vi "Autonomous Independent.vi"() -> ()   [LabVIEW 2016]
doc: "This VI is called when autonomous begins, and will automatically be terminated when autonomous ends. You can carry out timed or sensor driven robot movement independently without needing to return to the caller."
uses:
  <vilib>/Rock Robotics/WPI/Solenoid/WPI_SolenoidValue.ctl
  <vilib>/Rock Robotics/WPI/Utilities/WPI_GetSetVariantRefNum.vi
  <vilib>/Rock Robotics/Network Tables/NT Read String.vi
  <vilib>/Rock Robotics/Network Tables/NT Write Numeric Array.vi
  <vilib>/Rock Robotics/WPI/RobotDrive/WPI_RobotDriveArcadeDrive_Standard(NoSaturation).vi
  <vilib>/Rock Robotics/WPI/Solenoid/WPI_SolenoidSetEnum.vi
panel:
  out "encodervalue":dbl
  in  "Reset":bool
  out "Current Movement, for debugging":T1 {"Y Joystick Value" scale=1.0..-1.0; "X Joystick Value" scale=-1.0..1.0}
  in  "Array of robot movements":T2(array[cluster])=[{"X Joystick Value"=0.39393939393939403, "Y Joystick Value"=0.0, "Delay (sec)"=1.0, "Movement Name"="turn"}, {"X Joystick Value"=-0.3737373737373737, "Y Joystick Value"=0.0, "Delay (sec)"=1.0, "Movement Name"="turn back"}] {"Y Joystick Value" scale=1.0..-1.0; "X Joystick Value" scale=-1.0..1.0}
  # "Be sure to right-click and choose Data Operations>>Make Current Value default if you want to save the array values with the VI"
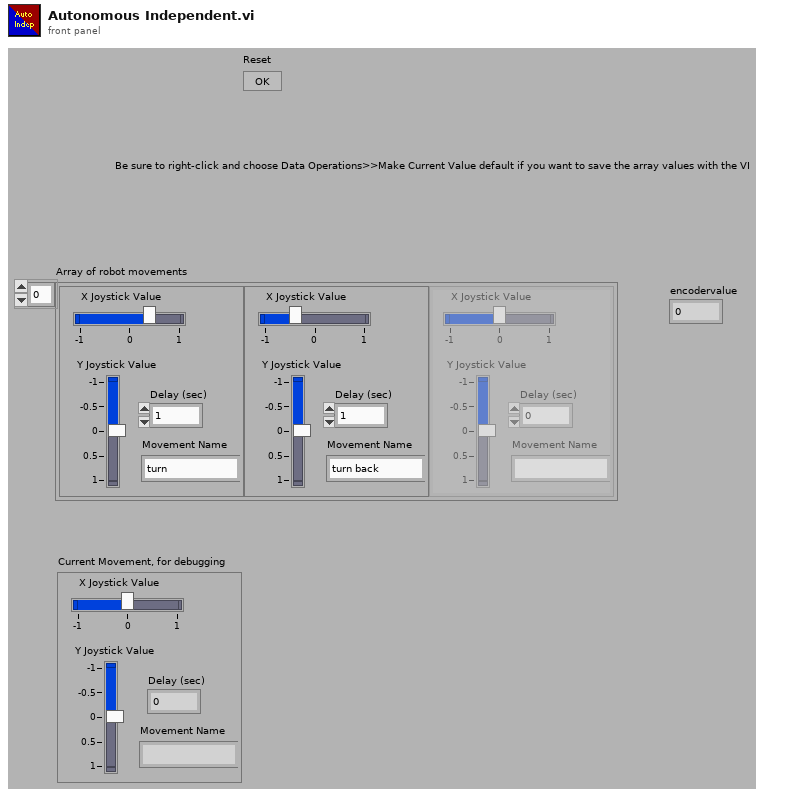
[diagram p1: front panel]
types:
  T1 = cluster{"X Joystick Value":dbl, "Y Joystick Value":dbl, "Delay (sec)":dbl, "Movement Name":string}
  T2 = cluster{"X Joystick Value":dbl, "Y Joystick Value":dbl, "Delay (sec)":dbl, "Movement Name":string}[]
  T3 = typedef "WPI_JoystickDevRef.ctl" = cluster{"Device":T4}
  T4 = typedef "WPI_JoystickDeviceEnum.ctl" = enum16{"USB 0", "USB 1", "USB 2", "USB 3", "USB 4", "USB 5"}
  T5 = typedef "WPI_EncoderDevRef.ctl" = cluster{"DevStatus":errorcluster, "EncoderIndex":T6, "CounterIndex":T7, "DistancePerCount":dbl, "Decoding Type":T8}
  T6 = typedef "FPGA_EncoderIdx.ctl" = enum8{"Enc 0", "Enc 1", "Enc 2", "Enc 3", "Enc 4", "Enc 5", "Enc 6", "Enc 7", "Invalid"}
  T7 = typedef "FPGA_CounterCtrSystemIndex.ctl" = enum8{"Ctr 0", "Ctr 1", "Ctr 2", "Ctr 3", "Ctr 4", "Ctr 5", "Ctr 6", "Ctr 7", "Invalid"}
  T8 = typedef "WPI_EncoderType.ctl" = enum16{"1x", "2x", "4x"}
  T9 = typedef "WPI_GyroDevRef.ctl" = cluster{"DevStatus":errorcluster, "Analog Channel":T10, "Offset":dbl, "Gain (VoltsPerDegree/Second)":dbl, "Gyro Type":enum16{"Analog", "XRS450"}, "Handle":i32, "SPI Bus":T11, "Device Found":bool, "Sample Rate":dbl, "Calibrate On Open":bool}
  T10 = typedef "FPGA_AIChannel.ctl" = enum8{"AI 0", "AI 1", "AI 2", "AI 3", "AI MXP 0", "AI MXP 1", "AI MXP 2", "AI MXP 3", "Invalid"}
  T11 = typedef "spi_bus.ctl" = enum16{"SPI On-Board, CS0", "SPI On-Board, CS1", "SPI On-Board, CS2", "SPI On-Board, CS3", "SPI MXP", "Invalid"}
  T12 = typedef "WPI_RobotDriveDevRef.ctl" = cluster{"DevStatus":errorcluster, "Motors[]":T13[], "Square Inputs":bool, "Max Output":dbl}
  T13 = typedef "WPI_MotorControlDeviceRef.ctl" = cluster{"DeviceStatus":errorcluster, "Type":T14, "PWM":cluster{"PWM Channel":T15, "DeadBand":T16}, "CAN":cluster{"Device Number":u8, "SetOutput VI Ref":variant, "GetOutput VI Ref":variant, "Enable VI Ref":variant, "Disable VI Ref":variant, "Data":variant}, "Invert":bool}
  T14 = typedef "WPI_MotorControlType.ctl" = enum16{"PWM", "CAN"}
  T15 = typedef "FPGA_DIOPWMChannel.ctl" = enum8{"PWM 0", "PWM 1", "PWM 2", "PWM 3", "PWM 4", "PWM 5", "PWM 6", "PWM 7", "PWM 8", "PWM 9", "PWM MXP 0", "PWM MXP 1", "PWM MXP 2", "PWM MXP 3", "PWM MXP 4", "PWM MXP 5", "PWM MXP 6", "PWM MXP 7", "PWM MXP 8", "PWM MXP 9", "Invalid"}
  T16 = typedef "WPI_PWMDeadband.ctl" = cluster{"Name":string, "maxPositivePwm":i32, "minPositivePwm":i32, "centerPwm":i32, "maxNegativePwm":i32, "minNegativePwm":i32, "angularRange":u16}
  T17 = typedef "WPI_SolenoidValue.ctl" = enum16{"Off", "On", "Forward", "Reverse"}
  T18 = typedef "WPI_SolenoidDevRef.ctl" = cluster{"DevStatus":errorcluster, "Pneumatics Control Module":u8, "Forward Solenoid Channel":T19, "Reverse Solenoid Channel":T19}
  T19 = typedef "WPI_SolenoidChannel.ctl" = enum8{"Solenoid 0", "Solenoid 1", "Solenoid 2", "Solenoid 3", "Solenoid 4", "Solenoid 5", "Solenoid 6", "Solenoid 7", "Invalid"}
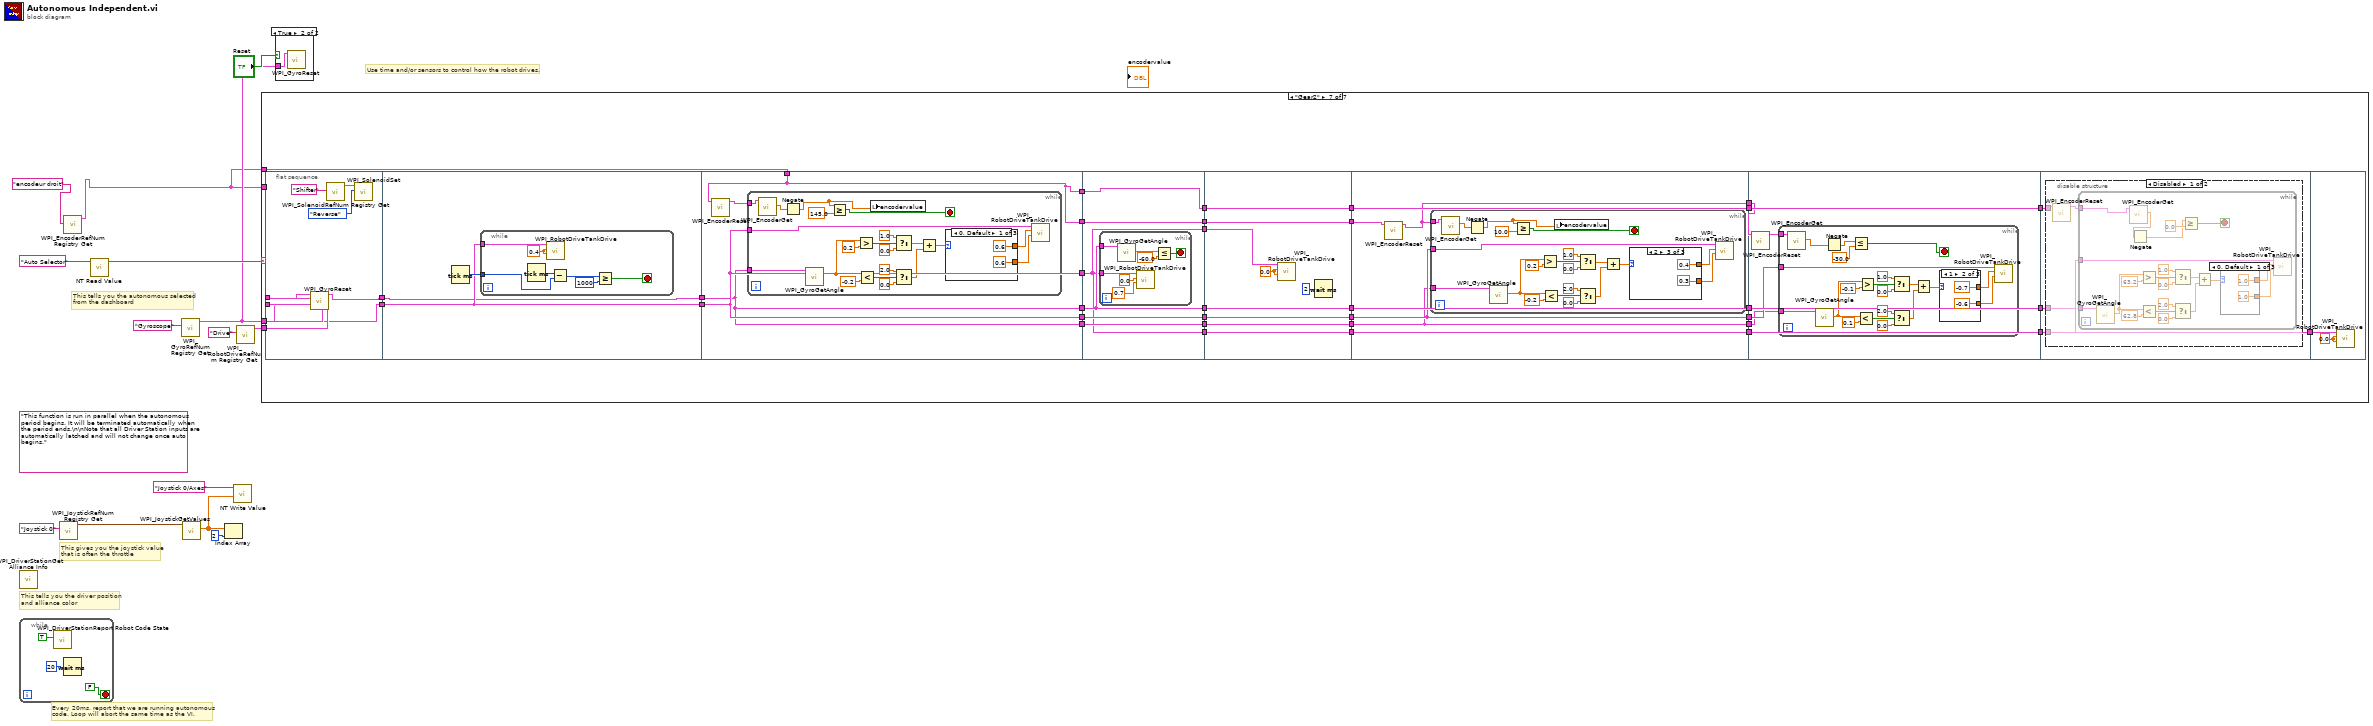
[diagram p0: block diagram]
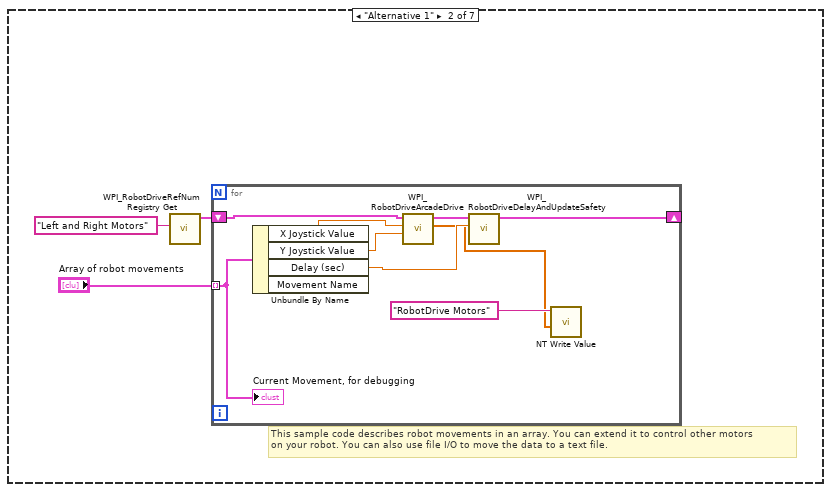
[diagram p4: hidden frame]
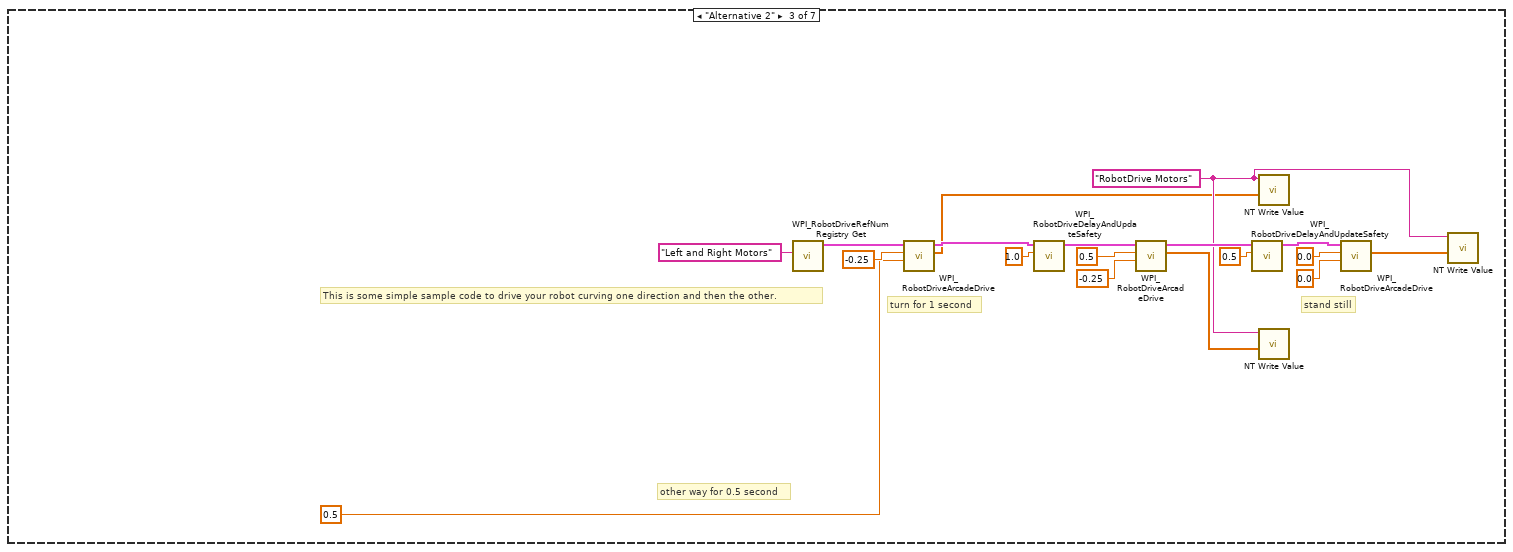
[diagram p5: hidden frame]
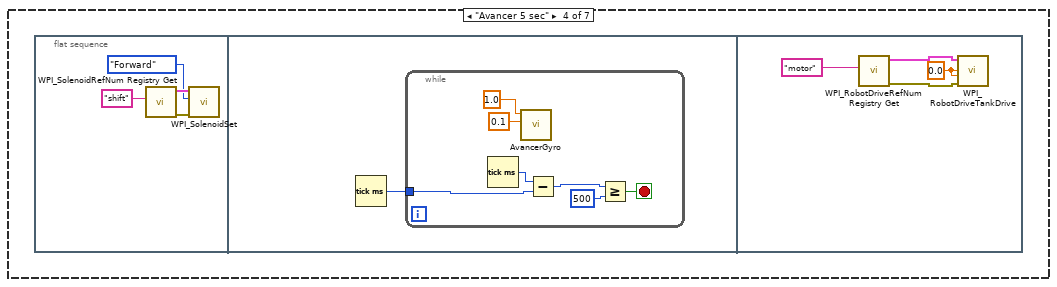
[diagram p6: hidden frame]
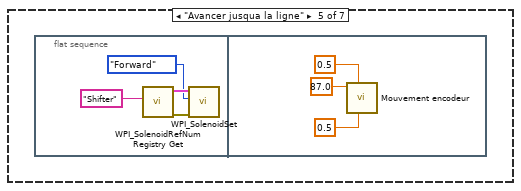
[diagram p7: hidden frame]
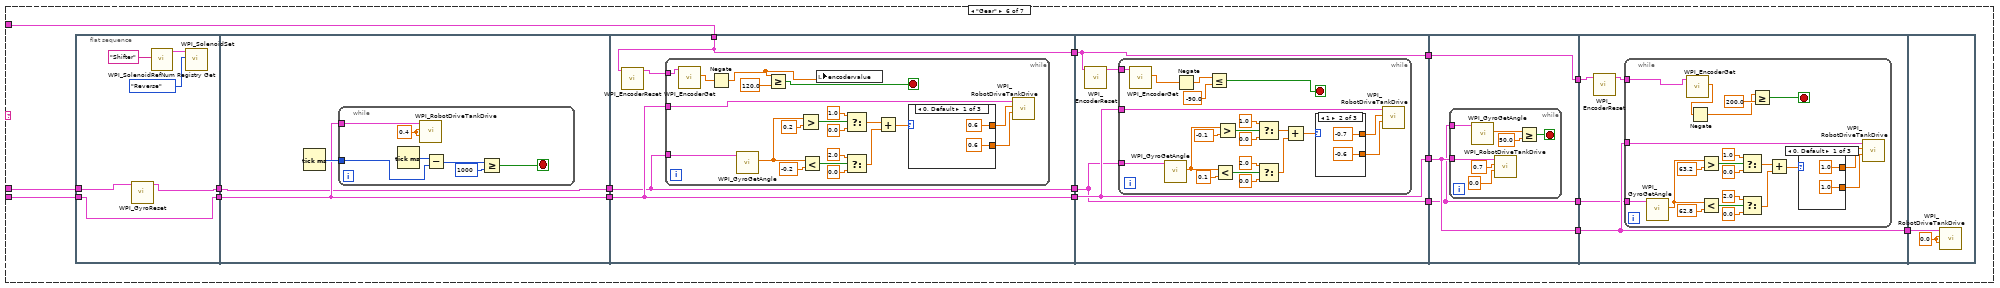
[diagram p8: hidden frame]
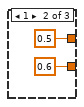
[diagram p9: hidden frame]
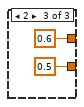
[diagram p10: hidden frame]
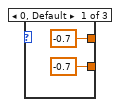
[diagram p11: hidden frame]
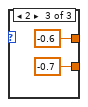
[diagram p12: hidden frame]
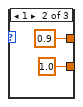
[diagram p13: hidden frame]
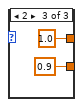
[diagram p14: hidden frame]
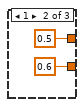
[diagram p15: hidden frame]
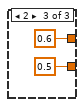
[diagram p16: hidden frame]
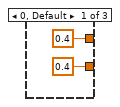
[diagram p17: hidden frame]
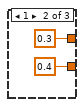
[diagram p18: hidden frame]
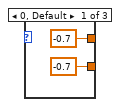
[diagram p19: hidden frame]
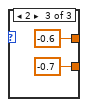
[diagram p20: hidden frame]
diagram:
  (unwired) "This function is run in parallel when the autonomous period begins. It will be terminated automatically when the period ends.\n\nNote that all Driver Station inputs are automatically latched and will not change once auto begins."
  # "This tells you the autonomous selected\nfrom the dashboard"
  # "Every 20ms, report that we are running autonomous\ncode. Loop will abort the same time as the VI."
  # "This gives you the joystick value\nthat is often the throttle"
  # "Use time and/or sensors to control how the robot drives."
  # "This tells you the driver position\nand alliance color"
  n1 = call <vilib>:"WPI_DriverStationGet Alliance Info.vi"() -> ()  [unwired: 12 out]
  n2 = while {
    stop <- FALSE stop-if-true
    n3 = call <vilib>:"WPI_DriverStationReport Robot Code State.vi"("Autonomous"=TRUE) -> ()  [unwired: 10 in, 1 out]
    n4 = Wait (ms)(milliseconds to wait=u32 20) -> ()  [unwired: 1 out]
  }
  n5 = call <vilib>:"WPI_JoystickRefNum Registry Get.vi"("refnum name"="Joystick 0") -> ("JoystickDevRef"=w13:T3)  [unwired: 1 in, 9 out]
  n6 = call <vilib>:"WPI_EncoderRefNum Registry Get.vi"("refnum name"="encodeur droit") -> ("EncoderDevRef"=w1:T5)  [unwired: 9 in, 1 out]
  n7 = call-poly <vilib>:"NT Read Value.vi"("Name"="Auto Selector") -> ("String"=w8:string)  [unwired: 9 in, 1 out]
  n8 = call <vilib>:"WPI_GyroRefNum Registry Get.vi"("refnum name"="Gyroscope") -> ("GyroDevRef"=w3:T9)  [unwired: 9 in, 1 out]
  n9 = call <vilib>:"WPI_JoystickGetValues.vi"("JoystickDevRef"=w13) -> ("Axes"=w10:dbl[])  [unwired: 6 in, 4 out]
  n10 = Index Array(array=w10, index=2) -> ()  [unwired: 1 out]
  n11 = call-poly <vilib>:"NT Write Value.vi"("Numeric Array"=w10, "Name"="Joystick 0/Axes") -> ()  [unwired: 9 in, 1 out]
  n12 = call <vilib>:"WPI_RobotDriveRefNum Registry Get.vi"("refnum name"="Drive") -> ("RobotDriveDevRef"=w6:T12)  [unwired: 9 in, 1 out]
  n13 = case shown="\"Gear2\"" w8 {
    tunnel: w6 -> [_ _ _ _ _ w87 w238]
    tunnel: w3 -> [_ _ _ _ _ w81 w239]
    tunnel: w1 -> [_ _ _ _ _ w74 _]
    tunnel: w1 -> [_ _ _ _ _ _ w237]
    frame Default {
      # "You can put your main auto here, or you can right-click on the case and make any\nother frame be the default case."
      # "This is the frame that will execute if no selection is made, or if it is not recognized"
    }
    frame "Alternative 1" {
      # "This sample code describes robot movements in an array. You can extend it to control other motors\non your robot. You can also use file I/O to move the data to a text file."
      n14 = call <vilib>:"WPI_RobotDriveRefNum Registry Get.vi"("refnum name"="Left and Right Motors") -> ("RobotDriveDevRef"=w19:T12)  [unwired: 1 in, 9 out]
      n15 = for {
        shift-right: [w27] -> _
        shift-left: w19 -> [w28]
        tunnel: "Array of robot movements" -> [w23] mode=indexing
        n16 = Unbundle By Name(w23) -> ("X Joystick Value"=w26:dbl, "Y Joystick Value"=w25:dbl, "Delay (sec)"=w24:dbl)  [unwired: 1 out]
        n17 = call-poly <vilib>:"WPI_RobotDriveArcadeDrive.vi"("Y axis value"=w25, "X axis value"=w26, "RobotDriveDevRef"=w28) -> ("Motor Values"=w21:dbl[], "RobotDriveDevRef"=w29:T12)  [unwired: 1 in, 6 out]
        n18 = call <vilib>:"WPI_RobotDriveDelayAndUpdateSafety.vi"("Delay (s)"=w24, "RobotDriveDevRef"=w29) -> ("RobotDriveDevRef 2"=w27:T12)  [unwired: 8 in, 1 out]
        n19 = call-poly <vilib>:"NT Write Value.vi"("Numeric Array"=w21, "Name"="RobotDrive Motors") -> ()  [unwired: 9 in, 1 out]
        "Current Movement, for debugging" <- w23
      }
    }
    frame "Alternative 2" {
      w31 = "RobotDrive Motors" ("Name")
      # "This is some simple sample code to drive your robot curving one direction and then the other."
      # "stand still"
      # "other way for 0.5 second"
      # "turn for 1 second"
      n20 = call <vilib>:"WPI_RobotDriveRefNum Registry Get.vi"("refnum name"="Left and Right Motors") -> ("RobotDriveDevRef"=w47:T12)  [unwired: 1 in, 9 out]
      n21 = call-poly <vilib>:"WPI_RobotDriveArcadeDrive.vi"("Y axis value"=0.5 ("X axis value"), "X axis value"=-0.25, "RobotDriveDevRef"=w47) -> ("Motor Values"=w30:dbl[], "RobotDriveDevRef"=w40:T12)  [unwired: 1 in, 6 out]
      n22 = call <vilib>:"WPI_RobotDriveDelayAndUpdateSafety.vi"("Delay (s)"=1.0, "RobotDriveDevRef"=w40) -> ("RobotDriveDevRef 2"=w41:T12)  [unwired: 8 in, 1 out]
      n23 = call-poly <vilib>:"WPI_RobotDriveArcadeDrive.vi"("Y axis value"=-0.25 ("X axis value"), "X axis value"=0.5, "RobotDriveDevRef"=w41) -> ("Motor Values"=w32:dbl[], "RobotDriveDevRef"=w42:T12)  [unwired: 1 in, 6 out]
      n24 = call <vilib>:"WPI_RobotDriveDelayAndUpdateSafety.vi"("Delay (s)"=0.5, "RobotDriveDevRef"=w42) -> ("RobotDriveDevRef 2"=w43:T12)  [unwired: 8 in, 1 out]
      n25 = call-poly <vilib>:"NT Write Value.vi"("Numeric Array"=w30, "Name"=w31) -> ()  [unwired: 9 in, 1 out]
      n26 = call-poly <vilib>:"NT Write Value.vi"("Numeric Array"=w32, "Name"=w31) -> ()  [unwired: 9 in, 1 out]
      n27 = call-poly <vilib>:"WPI_RobotDriveArcadeDrive.vi"("Y axis value"=0.0 ("X axis value"), "X axis value"=0.0, "RobotDriveDevRef"=w43) -> ("Motor Values"=w33:dbl[])  [unwired: 1 in, 7 out]
      n28 = call-poly <vilib>:"NT Write Value.vi"("Numeric Array"=w33, "Name"=w31) -> ()  [unwired: 9 in, 1 out]
    }
    frame "Avancer 5 sec" {
      n29 = flat-sequence {
        frame #0 {
          n30 = call <vilib>:"WPI_SolenoidRefNum Registry Get.vi"("refnum name"="shift") -> ("error out"=w50:errorcluster, "SolenoidDevRef"=w49:T18)  [unwired: 9 in]
          n31 = call-poly <vilib>:"WPI_SolenoidSet.vi"("error in (no error)"=w50, "Value"=WPI_SolenoidValue."Forward", "SolenoidDevRef"=w49) -> ()  [unwired: 7 in, 2 out]
        }
        frame #1 {
          n32 = Tick Count (ms)() -> (millisecond timer value=w52:u32)
          n33 = while {
            tunnel: w52 -> [w56]
            stop <- w53 stop-if-true
            n34 = Tick Count (ms)() -> (millisecond timer value=w57:u32)
            n35 = call "AvancerGyro.vi"("Ajustement"=0.1, "Vitesse"=1.0) -> ()  [unwired: 10 in]
            n36 = Subtract(x=w57, y=w56) -> (x-y=w55:u32)
            n37 = Greater Or Equal?(x=w55, y=u32 500) -> (x >= y?=w53:bool)
          }
        }
        frame #2 {
          w63 = 0.0 ("Left axis value")
          n38 = call <vilib>:"WPI_RobotDriveRefNum Registry Get.vi"("refnum name"="motor") -> ("error out"=w62:errorcluster, "RobotDriveDevRef"=w61:T12)  [unwired: 9 in]
          n39 = call <vilib>:"WPI_RobotDriveTankDrive.vi"("error in (no error)"=w62, "Right axis value"=w63, "Left axis value"=w63, "RobotDriveDevRef"=w61) -> ()  [unwired: 5 in, 3 out]
        }
      }
    }
    frame "Avancer jusqua la ligne" {
      n40 = flat-sequence {
        frame #0 {
          n41 = call <vilib>:"WPI_SolenoidRefNum Registry Get.vi"("refnum name"="Shifter") -> ("error out"=w66:errorcluster, "SolenoidDevRef"=w65:T18)  [unwired: 9 in]
          n42 = call-poly <vilib>:"WPI_SolenoidSet.vi"("error in (no error)"=w66, "Value"=WPI_SolenoidValue."Forward", "SolenoidDevRef"=w65) -> ()  [unwired: 7 in, 2 out]
        }
        frame #1 {
          n43 = call "Mouvement encodeur.vi"("Vitesse initiale"=0.5, "Temps acceleration"=0.5, "Distance"=87.0) -> ()  [unwired: 9 in]
        }
      }
    }
    frame "Gear" {
      n44 = flat-sequence {
        tunnel: [w89] -> w85
        tunnel: w87 -> [w89]
        tunnel: [w88] -> w82
        tunnel: w81 -> [w90]
        tunnel: w85 -> [w95]
        tunnel: [w95] -> w84
        tunnel: [w94] -> w83
        tunnel: w82 -> [w94]
        tunnel: w84 -> [w107]
        tunnel: [w107] -> w86
        tunnel: w83 -> [w106]
        tunnel: [w106] -> w79
        tunnel: w74 -> [w105]
        tunnel: [w105] -> w73
        tunnel: w86 -> [w138]
        tunnel: [w138] -> w80
        tunnel: w79 -> [w137]
        tunnel: [w137] -> w78
        tunnel: w73 -> [w136]
        tunnel: [w136] -> w72
        tunnel: w80 -> [w168]
        tunnel: [w168] -> w77
        tunnel: w78 -> [w167]
        tunnel: [w167] -> w75
        tunnel: w72 -> [w166]
        tunnel: [w166] -> w71
        tunnel: w77 -> [w179]
        tunnel: [w179] -> w76
        tunnel: w75 -> [w178]
        tunnel: w71 -> [w177]
        tunnel: w76 -> [w207]
        frame #0 {
          n45 = call <vilib>:"WPI_GyroReset.vi"("GyroDevRef"=w90) -> ("GyroDevRef"=w88:T9)  [unwired: 9 in, 1 out]
          n46 = call <vilib>:"WPI_SolenoidRefNum Registry Get.vi"("refnum name"="Shifter") -> ("SolenoidDevRef"=w93:T18)  [unwired: 9 in, 1 out]
          n47 = call-poly <vilib>:"WPI_SolenoidSet.vi"("Value"=WPI_SolenoidValue."Reverse", "SolenoidDevRef"=w93) -> ()  [unwired: 8 in, 2 out]
        }
        frame #1 {
          n48 = Tick Count (ms)() -> (millisecond timer value=w96:u32)
          n49 = while {
            tunnel: w95 -> [w102]
            tunnel: w96 -> [w100]
            stop <- w97 stop-if-true
            w103 = 0.4 ("Left axis value")
            n50 = Tick Count (ms)() -> (millisecond timer value=w101:u32)
            n51 = call <vilib>:"WPI_RobotDriveTankDrive.vi"("Right axis value"=w103, "Left axis value"=w103, "RobotDriveDevRef"=w102) -> ()  [unwired: 6 in, 3 out]
            n52 = Subtract(x=w101, y=w100) -> (x-y=w99:u32)
            n53 = Greater Or Equal?(x=w99, y=u32 1000) -> (x >= y?=w97:bool)
          }
        }
        frame #2 {
          n54 = call <vilib>:"WPI_EncoderReset.vi"("EncoderDevRef"=w105) -> ("EncoderDevRef"=w104:T5)  [unwired: 9 in, 1 out]
          n55 = while {
            tunnel: w107 -> [w128]
            tunnel: w106 -> [w127]
            tunnel: w104 -> [w110]
            stop <- w111 stop-if-true
            n56 = call <vilib>:"WPI_EncoderGet.vi"("EncoderDevRef"=w110) -> ("Distance"=w109:dbl)  [unwired: 5 in, 5 out]
            n57 = Negate(x=w109) -> (-x=w108:dbl)
            n58 = call <vilib>:"WPI_GyroGetAngle.vi"("GyroDevRef"=w127) -> ("Angle"=w114:dbl)  [unwired: 6 in, 4 out]
            n59 = Greater Or Equal?(x=w108, y=120.0) -> (x >= y?=w111:bool)
            n60 = Greater?(x=w114, y=0.2) -> (0:w125:bool)
            n61 = Less?(x=w114, y=-0.2) -> (x < y?=w113:bool)
            n62 = local write "encodervalue"(w108) -> ()
            n63 = Select(t=1.0, s=w125, f=0.0) -> (s? t:f=w120:dbl)
            n64 = Select(t=2.0, s=w113, f=0.0) -> (s? t:f=w119:dbl)
            n65 = Add(x=w120, y=w119) -> (x+y=w118:dbl)
            n66 = case shown="0, Default" w118 {
              tunnel: [0.6 ("t") 0.5 ("t") 0.6 ("t")] -> w117
              tunnel: [0.6 ("f") 0.6 ("f") 0.5 ("f")] -> w116
              frame 0, Default {
              }
              frame 1 {
              }
              frame 2 {
              }
            }
            n67 = call <vilib>:"WPI_RobotDriveTankDrive.vi"("Right axis value"=w116, "Left axis value"=w117, "RobotDriveDevRef"=w128) -> ()  [unwired: 6 in, 3 out]
          }
        }
        frame #3 {
          n68 = call <vilib>:"WPI_EncoderReset.vi"("EncoderDevRef"=w136) -> ("EncoderDevRef"=w135:T5)  [unwired: 9 in, 1 out]
          n69 = while {
            tunnel: w138 -> [w147]
            tunnel: w137 -> [w144]
            tunnel: w135 -> [w141]
            stop <- w142 stop-if-true
            n70 = call <vilib>:"WPI_EncoderGet.vi"("EncoderDevRef"=w141) -> ("Distance"=w140:dbl)  [unwired: 5 in, 5 out]
            n71 = call <vilib>:"WPI_GyroGetAngle.vi"("GyroDevRef"=w144) -> ("Angle"=w158:dbl)  [unwired: 6 in, 4 out]
            n72 = Negate(x=w140) -> (-x=w139:dbl)
            n73 = Less Or Equal?(x=w139, y=-90.0) -> (x <= y?=w142:bool)
            n74 = Less?(x=w158, y=0.1) -> (x < y?=w159:bool)
            n75 = Greater?(x=w158, y=-0.1) -> (0:w149:bool)
            n76 = Select(t=1.0, s=w149, f=0.0) -> (s? t:f=w154:dbl)
            n77 = Select(t=2.0, s=w159, f=0.0) -> (s? t:f=w155:dbl)
            n78 = Add(x=w154, y=w155) -> (x+y=w156:dbl)
            n79 = case shown="1" w156 {
              tunnel: [-0.7 ("t") -0.7 ("t") -0.6 ("t")] -> w146
              tunnel: [-0.7 ("f") -0.6 ("f") -0.7 ("f")] -> w145
              frame 0, Default {
              }
              frame 1 {
              }
              frame 2 {
              }
            }
            n80 = call <vilib>:"WPI_RobotDriveTankDrive.vi"("Right axis value"=w145, "Left axis value"=w146, "RobotDriveDevRef"=w147) -> ()  [unwired: 6 in, 3 out]
          }
        }
        frame #4 {
          n81 = while {
            tunnel: w167 -> [w172]
            tunnel: w168 -> [w169]
            stop <- w173 stop-if-true
            n82 = call <vilib>:"WPI_GyroGetAngle.vi"("GyroDevRef"=w172) -> ("Angle"=w175:dbl)  [unwired: 6 in, 4 out]
            n83 = call <vilib>:"WPI_RobotDriveTankDrive.vi"("Right axis value"=0.0, "Left axis value"=0.7, "RobotDriveDevRef"=w169) -> ()  [unwired: 6 in, 3 out]
            n84 = Greater Or Equal?(x=w175, y=50.0) -> (x >= y?=w173:bool)
          }
        }
        frame #5 {
          n85 = call <vilib>:"WPI_EncoderReset.vi"("EncoderDevRef"=w177) -> ("EncoderDevRef"=w176:T5)  [unwired: 9 in, 1 out]
          n86 = while {
            tunnel: w179 -> [w200]
            tunnel: w178 -> [w198]
            tunnel: w176 -> [w182]
            stop <- w199 stop-if-true
            n87 = call <vilib>:"WPI_GyroGetAngle.vi"("GyroDevRef"=w198) -> ("Angle"=w185:dbl)  [unwired: 6 in, 4 out]
            n88 = call <vilib>:"WPI_EncoderGet.vi"("EncoderDevRef"=w182) -> ("Distance"=w181:dbl)  [unwired: 5 in, 5 out]
            n89 = Negate(x=w181) -> (-x=w180:dbl)
            n90 = Greater?(x=w185, y=63.2) -> (0:w196:bool)
            n91 = Less?(x=w185, y=62.8) -> (x < y?=w184:bool)
            n92 = Select(t=1.0, s=w196, f=0.0) -> (s? t:f=w191:dbl)
            n93 = Select(t=2.0, s=w184, f=0.0) -> (s? t:f=w190:dbl)
            n94 = Greater Or Equal?(x=w180, y=200.0) -> (x >= y?=w199:bool)
            n95 = Add(x=w191, y=w190) -> (x+y=w189:dbl)
            n96 = case shown="0, Default" w189 {
              tunnel: [1.0 ("t") 0.9 ("t") 1.0 ("t")] -> w188
              tunnel: [1.0 ("f") 1.0 ("f") 0.9 ("f")] -> w187
              frame 0, Default {
              }
              frame 1 {
              }
              frame 2 {
              }
            }
            n97 = call <vilib>:"WPI_RobotDriveTankDrive.vi"("Right axis value"=w187, "Left axis value"=w188, "RobotDriveDevRef"=w200) -> ()  [unwired: 6 in, 3 out]
          }
        }
        frame #6 {
          w208 = 0.0 ("Left axis value")
          n98 = call <vilib>:"WPI_RobotDriveTankDrive.vi"("Right axis value"=w208, "Left axis value"=w208, "RobotDriveDevRef"=w207) -> ()  [unwired: 6 in, 3 out]
        }
      }
    }
    frame "Gear2" {
      n99 = flat-sequence {
        tunnel: [w246] -> w244
        tunnel: w238 -> [w246]
        tunnel: [w245] -> w243
        tunnel: w239 -> [w247]
        tunnel: w244 -> [w252]
        tunnel: [w252] -> w242
        tunnel: [w251] -> w241
        tunnel: w243 -> [w251]
        tunnel: w242 -> [w263]
        tunnel: [w263] -> w236
        tunnel: w241 -> [w262]
        tunnel: [w262] -> w235
        tunnel: w237 -> [w261]
        tunnel: [w261] -> w234
        tunnel: [w263] -> w233
        tunnel: [w262] -> w232
        tunnel: [w261] -> w231
        tunnel: w236 -> [w292]
        tunnel: [w292] -> w221
        tunnel: w235 -> [w297]
        tunnel: [w297] -> w219
        tunnel: [w296] -> w217
        tunnel: w234 -> [w296]
        tunnel: [w295] -> w215
        tunnel: w233 -> [w295]
        tunnel: [w294] -> w213
        tunnel: w232 -> [w294]
        tunnel: [w293] -> w211
        tunnel: w231 -> [w293]
        tunnel: [w292] -> w209
        tunnel: w221 -> [w313]
        tunnel: [w313] -> w220
        tunnel: w219 -> [w312]
        tunnel: [w312] -> w218
        tunnel: w217 -> [w311]
        tunnel: [w311] -> w216
        tunnel: w215 -> [w310]
        tunnel: [w310] -> w214
        tunnel: w213 -> [w309]
        tunnel: [w309] -> w212
        tunnel: w211 -> [w308]
        tunnel: [w308] -> w210
        tunnel: w209 -> [w306]
        tunnel: w220 -> [w320]
        tunnel: [w320] -> w230
        tunnel: w218 -> [w319]
        tunnel: [w319] -> w228
        tunnel: w216 -> [w318]
        tunnel: [w318] -> w226
        tunnel: w214 -> [w317]
        tunnel: w212 -> [w316]
        tunnel: w210 -> [w314]
        tunnel: [w317] -> w224
        tunnel: [w316] -> w223
        tunnel: [w315] -> w222
        tunnel: w230 -> [w354]
        tunnel: [w354] -> w229
        tunnel: w228 -> [w353]
        tunnel: [w353] -> w227
        tunnel: w226 -> [w352]
        tunnel: [w352] -> w225
        tunnel: w224 -> [w350]
        tunnel: w223 -> [w349]
        tunnel: w222 -> [w348]
        tunnel: w229 -> [w384]
        tunnel: [w384] -> w240
        tunnel: w227 -> [w383]
        tunnel: w225 -> [w382]
        tunnel: w240 -> [w416]
        frame #0 {
          n100 = call <vilib>:"WPI_GyroReset.vi"("GyroDevRef"=w247) -> ("GyroDevRef"=w245:T9)  [unwired: 9 in, 1 out]
          n101 = call <vilib>:"WPI_SolenoidRefNum Registry Get.vi"("refnum name"="Shifter") -> ("SolenoidDevRef"=w250:T18)  [unwired: 9 in, 1 out]
          n102 = call-poly <vilib>:"WPI_SolenoidSet.vi"("Value"=WPI_SolenoidValue."Reverse", "SolenoidDevRef"=w250) -> ()  [unwired: 8 in, 2 out]
        }
        frame #1 {
          n103 = Tick Count (ms)() -> (millisecond timer value=w253:u32)
          n104 = while {
            tunnel: w252 -> [w259]
            tunnel: w253 -> [w257]
            stop <- w254 stop-if-true
            w260 = 0.4 ("Left axis value")
            n105 = Tick Count (ms)() -> (millisecond timer value=w258:u32)
            n106 = call <vilib>:"WPI_RobotDriveTankDrive.vi"("Right axis value"=w260, "Left axis value"=w260, "RobotDriveDevRef"=w259) -> ()  [unwired: 6 in, 3 out]
            n107 = Subtract(x=w258, y=w257) -> (x-y=w256:u32)
            n108 = Greater Or Equal?(x=w256, y=u32 1000) -> (x >= y?=w254:bool)
          }
        }
        frame #2 {
          n109 = call <vilib>:"WPI_EncoderReset.vi"("EncoderDevRef"=w261) -> ("EncoderDevRef"=w264:T5)  [unwired: 9 in, 1 out]
          n110 = while {
            tunnel: w263 -> [w285]
            tunnel: w262 -> [w284]
            tunnel: w264 -> [w267]
            stop <- w268 stop-if-true
            n111 = call <vilib>:"WPI_EncoderGet.vi"("EncoderDevRef"=w267) -> ("Distance"=w266:dbl)  [unwired: 5 in, 5 out]
            n112 = Negate(x=w266) -> (-x=w265:dbl)
            n113 = call <vilib>:"WPI_GyroGetAngle.vi"("GyroDevRef"=w284) -> ("Angle"=w271:dbl)  [unwired: 6 in, 4 out]
            n114 = Greater Or Equal?(x=w265, y=145.0) -> (x >= y?=w268:bool)
            n115 = Greater?(x=w271, y=0.2) -> (0:w282:bool)
            n116 = Less?(x=w271, y=-0.2) -> (x < y?=w270:bool)
            n117 = local write "encodervalue"(w265) -> ()
            n118 = Select(t=1.0, s=w282, f=0.0) -> (s? t:f=w277:dbl)
            n119 = Select(t=2.0, s=w270, f=0.0) -> (s? t:f=w276:dbl)
            n120 = Add(x=w277, y=w276) -> (x+y=w275:dbl)
            n121 = case shown="0, Default" w275 {
              tunnel: [0.6 ("t") 0.5 ("t") 0.6 ("t")] -> w274
              tunnel: [0.6 ("f") 0.6 ("f") 0.5 ("f")] -> w273
              frame 0, Default {
              }
              frame 1 {
              }
              frame 2 {
              }
            }
            n122 = call <vilib>:"WPI_RobotDriveTankDrive.vi"("Right axis value"=w273, "Left axis value"=w274, "RobotDriveDevRef"=w285) -> ()  [unwired: 6 in, 3 out]
          }
        }
        frame #3 {
          n123 = while {
            tunnel: w297 -> [w301]
            tunnel: w292 -> [w298]
            stop <- w302 stop-if-true
            n124 = call <vilib>:"WPI_GyroGetAngle.vi"("GyroDevRef"=w301) -> ("Angle"=w304:dbl)  [unwired: 6 in, 4 out]
            n125 = call <vilib>:"WPI_RobotDriveTankDrive.vi"("Right axis value"=0.7, "Left axis value"=0.0, "RobotDriveDevRef"=w298) -> ()  [unwired: 6 in, 3 out]
            n126 = Less Or Equal?(x=w304, y=-60.0) -> (x <= y?=w302:bool)
          }
        }
        frame #4 {
          w307 = 0.0 ("Left axis value")
          n127 = call <vilib>:"WPI_RobotDriveTankDrive.vi"("Right axis value"=w307, "Left axis value"=w307, "RobotDriveDevRef"=w306) -> ()  [unwired: 6 in, 3 out]
          n128 = Wait (ms)(milliseconds to wait=u32 2) -> ()  [unwired: 1 out]
        }
        frame #5 {
          n129 = call <vilib>:"WPI_EncoderReset.vi"("EncoderDevRef"=w314) -> ("EncoderDevRef"=w315:T5)  [unwired: 9 in, 1 out]
          n130 = while {
            tunnel: w317 -> [w341]
            tunnel: w316 -> [w340]
            tunnel: w315 -> [w323]
            stop <- w324 stop-if-true
            n131 = call <vilib>:"WPI_EncoderGet.vi"("EncoderDevRef"=w323) -> ("Distance"=w322:dbl)  [unwired: 5 in, 5 out]
            n132 = Negate(x=w322) -> (-x=w321:dbl)
            n133 = call <vilib>:"WPI_GyroGetAngle.vi"("GyroDevRef"=w340) -> ("Angle"=w327:dbl)  [unwired: 6 in, 4 out]
            n134 = Greater Or Equal?(x=w321, y=10.0) -> (x >= y?=w324:bool)
            n135 = Greater?(x=w327, y=0.2) -> (0:w338:bool)
            n136 = Less?(x=w327, y=-0.2) -> (x < y?=w326:bool)
            n137 = local write "encodervalue"(w321) -> ()
            n138 = Select(t=1.0, s=w338, f=0.0) -> (s? t:f=w333:dbl)
            n139 = Select(t=2.0, s=w326, f=0.0) -> (s? t:f=w332:dbl)
            n140 = Add(x=w333, y=w332) -> (x+y=w331:dbl)
            n141 = case shown="2" w331 {
              tunnel: [0.4 ("t") 0.3 ("t") 0.4 ("t")] -> w330
              tunnel: [0.4 ("f") 0.4 ("f") 0.3 ("f")] -> w329
              frame 0, Default {
              }
              frame 1 {
              }
              frame 2 {
              }
            }
            n142 = call <vilib>:"WPI_RobotDriveTankDrive.vi"("Right axis value"=w329, "Left axis value"=w330, "RobotDriveDevRef"=w341) -> ()  [unwired: 6 in, 3 out]
          }
        }
        frame #6 {
          n143 = call <vilib>:"WPI_EncoderReset.vi"("EncoderDevRef"=w348) -> ("EncoderDevRef"=w351:T5)  [unwired: 9 in, 1 out]
          n144 = while {
            tunnel: w350 -> [w363]
            tunnel: w349 -> [w360]
            tunnel: w351 -> [w357]
            stop <- w358 stop-if-true
            n145 = call <vilib>:"WPI_EncoderGet.vi"("EncoderDevRef"=w357) -> ("Distance"=w356:dbl)  [unwired: 5 in, 5 out]
            n146 = call <vilib>:"WPI_GyroGetAngle.vi"("GyroDevRef"=w360) -> ("Angle"=w374:dbl)  [unwired: 6 in, 4 out]
            n147 = Negate(x=w356) -> (-x=w355:dbl)
            n148 = Less Or Equal?(x=w355, y=-30.0) -> (x <= y?=w358:bool)
            n149 = Less?(x=w374, y=0.1) -> (x < y?=w375:bool)
            n150 = Greater?(x=w374, y=-0.1) -> (0:w365:bool)
            n151 = Select(t=1.0, s=w365, f=0.0) -> (s? t:f=w370:dbl)
            n152 = Select(t=2.0, s=w375, f=0.0) -> (s? t:f=w371:dbl)
            n153 = Add(x=w370, y=w371) -> (x+y=w372:dbl)
            n154 = case shown="1" w372 {
              tunnel: [-0.7 ("t") -0.7 ("t") -0.6 ("t")] -> w362
              tunnel: [-0.7 ("f") -0.6 ("f") -0.7 ("f")] -> w361
              frame 0, Default {
              }
              frame 1 {
              }
              frame 2 {
              }
            }
            n155 = call <vilib>:"WPI_RobotDriveTankDrive.vi"("Right axis value"=w361, "Left axis value"=w362, "RobotDriveDevRef"=w363) -> ()  [unwired: 6 in, 3 out]
          }
        }
        frame #7 {
          n156 = disable-structure shown="Disabled" {
            disable-tunnel: w384 -> [w388 _]
            disable-tunnel: w383 -> [w387 _]
            disable-tunnel: w382 -> [w386 _]
            frame Disabled {
              n157 = call <vilib>:"WPI_EncoderReset.vi"("EncoderDevRef"=w386) -> ("EncoderDevRef"=w385:T5)  [unwired: 9 in, 1 out]
              n158 = while {
                tunnel: w388 -> [w409]
                tunnel: w387 -> [w407]
                tunnel: w385 -> [w391]
                stop <- w408 stop-if-true
                n159 = call <vilib>:"WPI_GyroGetAngle.vi"("GyroDevRef"=w407) -> ("Angle"=w394:dbl)  [unwired: 6 in, 4 out]
                n160 = call <vilib>:"WPI_EncoderGet.vi"("EncoderDevRef"=w391) -> ("Distance"=w390:dbl)  [unwired: 5 in, 5 out]
                n161 = Negate(x=w390) -> (-x=w389:dbl)
                n162 = Greater?(x=w394, y=63.2) -> (0:w405:bool)
                n163 = Less?(x=w394, y=62.8) -> (x < y?=w393:bool)
                n164 = Select(t=1.0, s=w405, f=0.0) -> (s? t:f=w400:dbl)
                n165 = Select(t=2.0, s=w393, f=0.0) -> (s? t:f=w399:dbl)
                n166 = Greater Or Equal?(x=w389, y=0.0) -> (x >= y?=w408:bool)
                n167 = Add(x=w400, y=w399) -> (x+y=w398:dbl)
                n168 = case shown="0, Default" w398 {
                  tunnel: [1.0 ("t") 0.9 ("t") 1.0 ("t")] -> w397
                  tunnel: [1.0 ("f") 1.0 ("f") 0.9 ("f")] -> w396
                  frame 0, Default {
                  }
                  frame 1 {
                  }
                  frame 2 {
                  }
                }
                n169 = call <vilib>:"WPI_RobotDriveTankDrive.vi"("Right axis value"=w396, "Left axis value"=w397, "RobotDriveDevRef"=w409) -> ()  [unwired: 6 in, 3 out]
              }
            }
            frame Enabled {
            }
          }
        }
        frame #8 {
          w417 = 0.0 ("Left axis value")
          n170 = call <vilib>:"WPI_RobotDriveTankDrive.vi"("Right axis value"=w417, "Left axis value"=w417, "RobotDriveDevRef"=w416) -> ()  [unwired: 6 in, 3 out]
        }
      }
    }
  }
  n171 = case shown="True" "Reset" {
    tunnel: w3 -> [_ w418]
    frame False {
    }
    frame True {
      n172 = call <vilib>:"WPI_GyroReset.vi"("GyroDevRef"=w418) -> ()  [unwired: 9 in, 2 out]
    }
  }
